vi "MatchRegExSubstrArrayByName.vi"(5 "capture name":string[](array[string]), 7 "Options":cluster{"Compile":u32, "Match":u32} {"Match" format="%.0x"; "Compile" format="%.0x"}, 8 "error in":errorcluster, 9 "offset (0)":u64, 10 "search pattern":string, 11 "string":string) -> (0 "error out":errorcluster, 2 "substrings":string[](array[string]), 4 "NextStartOffset":i32, 6 "ContinueMatch?":bool)   [LabVIEW 2021, in "libpcre2-8.lvlib"]
uses:
  libpcre2-8.lvlib
  Pcre2CompileError.vi
  Pcre2ErrorNull.vi
  Pcre2LibError.vi
  Pcre2FnkCallError.vi
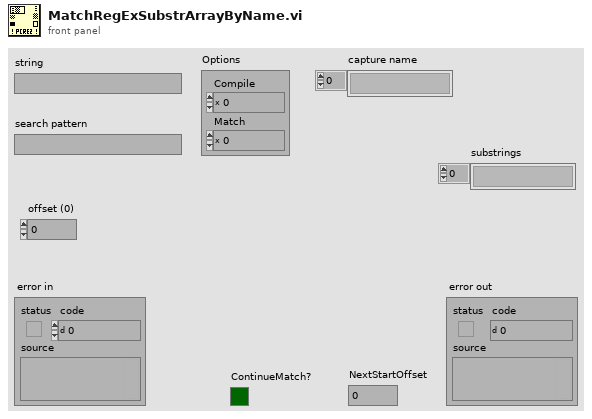
[diagram p1: front panel]
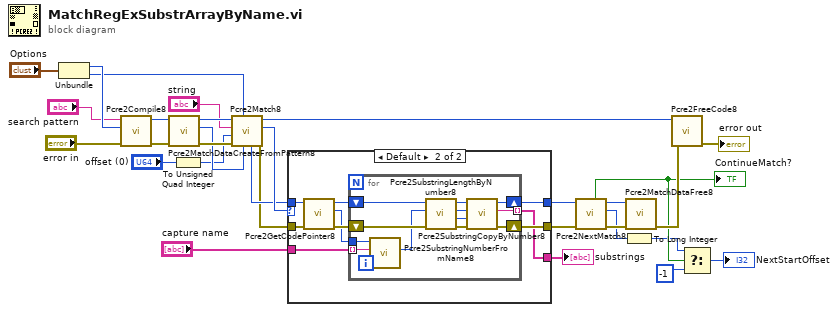
[diagram p0: block diagram]
diagram:
  n1 = Unbundle("Options") -> ("Compile"=w22:u32, "Match"=w21:u32)
  n2 = call "Pcre2Compile8.vi"("error in"="error in", "Options"=w22, "Pattern"="search pattern") -> ("error out"=w28:errorcluster, "pCode"=w27:u64)  [unwired: 7 in]
  n3 = call "Pcre2MatchDataCreateFromPattern8.vi"("error in"=w28, "pCode"=w27) -> ("error out"=w29:errorcluster, "pMatchData"=w20:u64, "pCode"=w30:u64)  [unwired: 7 in]
  n4 = To Unsigned Quad Integer(1:"offset (0)") -> (0:w5:u64)
  n5 = call "Pcre2Match8.vi"("pMatchData"=w20, "Options"=w21, "error in"=w29, "StartOffset"=w5, "Subject"="string", "pCode"=w30) -> ("error out"=w7:errorcluster, "MatchResult"=w9:i32, "pCode"=w26:u64, "pMatchData"=w8:u64)  [unwired: 2 in]
  n6 = case shown="Default" w9 {
    tunnel: w8 -> [w32 w38]
    tunnel: [_ w33] -> w14
    tunnel: [w32 w41] -> w13
    tunnel: "capture name" -> [_ w39]
    tunnel: w7 -> [w31 w37]
    tunnel: [w31 w40] -> w11
    frame ..-1 {
    }
    frame Default {
      n7 = call "Pcre2GetCodePointer8.vi"("error in"=w37, "pMatchData"=w38) -> ("error out"=w35:errorcluster, "pCode"=w34:u64, "pMatchData"=w36:u64)  [unwired: 7 in]
      n8 = for {
        tunnel: w39 -> [w44] mode=indexing
        tunnel: [w45] -> w33 mode=indexing
        shift-right: [w53] -> w41
        shift-left: w36 -> [w51]
        shift-right: [w52] -> w40
        shift-left: w35 -> [w50]
        tunnel: w34 -> [w43]
        n9 = call "Pcre2SubstringNumberFromName8.vi"("Name"=w44, "pCode"=w43) -> ("Number"=w42:i32)  [unwired: 7 in, 2 out]
        n10 = call "Pcre2SubstringLengthByNumber8.vi"("error in"=w50, "Number"=w42, "pMatchData"=w51) -> ("error out"=w49:errorcluster, "Length"=w47:u64, "Number"=w46:i32, "pMatchData"=w48:u64)  [unwired: 5 in]
        n11 = call "Pcre2SubstringCopyByNumber8.vi"("error in"=w49, "Length"=w47, "Number"=w46, "pMatchData"=w48) -> ("error out"=w52:errorcluster, "Substring"=w45:string, "pMatchData"=w53:u64)  [unwired: 5 in]
      }
    }
  }
  "substrings" <- w14
  n12 = call "Pcre2NextMatch8.vi"("error in"=w11, "pMatchData"=w13) -> ("error out"=w10:errorcluster, "NextStartOffset"=w6:u64, "pMatchData"=w12:u64, "ContinueMatch?"=w4:bool)  [unwired: 5 in, 1 out]
  "ContinueMatch?" <- w4
  n13 = To Long Integer(number=w6) -> (32bit integer=w1:i32)
  n14 = call "Pcre2MatchDataFree8.vi"("error in"=w10, "pMatchData"=w12) -> ("error out"=w25:errorcluster)  [unwired: 9 in]
  n15 = call "Pcre2FreeCode8.vi"("error in"=w25, "pCode"=w26) -> ("error out"=→"error out":errorcluster)  [unwired: 9 in]
  n16 = Select(t=w1, s=w4, f=-1) -> (s? t:f=→"NextStartOffset":i32)
